vi "NMRvmefull5.vi"() -> ()   [LabVIEW 2013]
uses:
  <vilib>/Utility/file.llb/Read From Spreadsheet File (DBL).vi
  <vilib>/Analysis/NI_AALBase.lvlib
panel:
  in  "Real/quad Q curve":bool=TRUE
  out "Temperature (C)":dbl(graph)=26.0
  out "+3V supply":dbl=3.026 format="%_4g"
  out "Temp (C)":dbl=26.0 format="%_4g"
  in  "RemovePed":bool=TRUE
  in  "IF / LOG Det":bool
  in  "Q curve file":string="realback213.txt"
  out "File name 2":string="C:\\users\\plm\\Desktop\\rssmt\\realback213.txt"
  in  "AutoBaseline":bool=TRUE
  out "RF OK":bool=TRUE
  out "Peak area (V-MHz)":sgl=0.047548737 format="%.5f"
  in  "Gauss Fit":bool=TRUE
  out "NMR Graph + Fit":cluster{cluster{dbl, "Numeric":dbl}[]}[](graph)=[{[{212.6, "Numeric"=-0.023529166666666664}, {212.60999999999999, "Numeric"=0.005982291666645268}, {212.62, "Numeric"=0.0036937500000235666}, {212.63, "Numeric"=-0.001994791666664122}, {212.64, "Numeric"=0.00021666666664931725}, {212.65, "Numeric"=-0.006471874999975841}, {212.66, "Numeric"=0.00913958333333801}, {212.67, "Numeric"=-0.005548958333346967}, {212.68, "Numeric"=0.01206250000002431}, {212.69, "Numeric"=0.004273958333339739}, {212.7, "Numeric"=0.00948541666665629}, {212.71, "Numeric"=0.006996875000024064}, {212.72, "Numeric"=0.010408333333341034}, {212.73, "Numeric"=-0.0007802083333407752}, {212.74, "Numeric"=-0.0026687500000218346}, {212.75, "Numeric"=0.00804270833334196}, {212.76, "Numeric"=-0.005945833333338348}, {212.77, "Numeric"=0.006565624999982199}, {212.78, "Numeric"=-0.014122916666657513}, {212.79, "Numeric"=0.004488541666663723}, {212.8, "Numeric"=-0.0026000000000141266}, {212.81, "Numeric"=-0.01418854166665745}, {212.82, "Numeric"=0.003322916666665406}, {212.82999999999998, "Numeric"=-0.0057656250000106815}, {212.84, "Numeric"=0.005045833333342235}, {212.85, "Numeric"=0.00045729166666663755}, {212.85999999999999, "Numeric"=0.009268749999992144}, {212.87, "Numeric"=0.0015802083333415066}, {212.88, "Numeric"=-0.0008083333333325294}, {212.89, "Numeric"=0.006903124999994543}, {212.9, "Numeric"=0.006914583333340364}, {212.91, "Numeric"=0.019626041666667912}, {212.92, "Numeric"=0.017537499999996535}, {212.93, "Numeric"=0.03184895833333881}, {212.94, "Numeric"=0.042160416666667914}, {212.95, "Numeric"=0.08397187499999814}, {212.96, "Numeric"=0.14308333333333687}, {212.97, "Numeric"=0.2796947916666675}, {212.98, "Numeric"=0.4758062499999993}, {212.99, "Numeric"=0.4924177083333319}, {213.0, "Numeric"=0.3697291666666667}, {213.01, "Numeric"=0.32994062500000004}, {213.02, "Numeric"=0.3085520833333343}, {213.03, "Numeric"=0.25276354166666554}, {213.04, "Numeric"=0.2412750000000005}, {213.05, "Numeric"=0.2554864583333362}, {213.06, "Numeric"=0.23649791666666387}, {213.07, "Numeric"=0.26220937500000036}, {213.08, "Numeric"=0.21542083333333772}, {213.09, "Numeric"=0.17623229166666188}, {213.1, "Numeric"=0.10804374999999992}, {213.11, "Numeric"=0.0878552083333388}, {213.12, "Numeric"=0.07366666666665944}, {213.13, "Numeric"=0.06387812499999908}, {213.14000000000001, "Numeric"=0.05268958333333953}, {213.15, "Numeric"=0.0238010416666566}, {213.16, "Numeric"=0.04101249999999778}, {213.17000000000002, "Numeric"=0.044323958333339825}, {213.18, "Numeric"=0.04973541666665334}, {213.19, "Numeric"=0.01754687499999609}, {213.2, "Numeric"=0.013558333333339938}, {213.21, "Numeric"=0.01546979166664969}, {213.22, "Numeric"=-0.0050187500000060045}, {213.23, "Numeric"=0.006992708333339413}, {213.24, "Numeric"=-0.004495833333314304}, {213.25, "Numeric"=-0.004484375000008534}, {213.26, "Numeric"=-0.020372916666661543}, {213.27, "Numeric"=-0.013161458333313683}, {213.28, "Numeric"=-0.02475000000001141}, {213.29, "Numeric"=-0.009238541666662908}, {213.3, "Numeric"=-0.003027083333313468}, {213.31, "Numeric"=-0.009215625000014757}, {213.32, "Numeric"=0.007595833333335376}, {213.33, "Numeric"=-0.01389270833331363}, {213.34, "Numeric"=-0.0015812500000184572}, {213.35, "Numeric"=-0.02236979166666679}, {213.36, "Numeric"=-0.005258333333314221}, {213.37, "Numeric"=-0.01264687500002265}, {213.38, "Numeric"=0.0028645833333306244}, {213.39000000000001, "Numeric"=0.003176041666684711}, {213.4, "Numeric"=-0.012812500000027156}]}, {[{212.6, "Numeric"=8.849236916727226e-16}, {212.60999999999999, "Numeric"=4.394384601054511e-15}, {212.62, "Numeric"=2.0985812753655877e-14}, {212.63, "Numeric"=9.638046352087863e-14}, {212.64, "Numeric"=4.2568438081885237e-13}, {212.65, "Numeric"=1.8080977585312592e-12}, {212.66, "Numeric"=7.385698722155563e-12}, {212.67, "Numeric"=2.9013275083294973e-11}, {212.68, "Numeric"=1.0960677793739773e-10}, {212.69, "Numeric"=3.9821127664234395e-10}, {212.7, "Numeric"=1.3913140959130146e-09}, {212.71, "Numeric"=4.674899766090939e-09}, {212.72, "Numeric"=1.5106188854084262e-08}, {212.73, "Numeric"=4.6943233797290934e-08}, {212.74, "Numeric"=1.4028995801745716e-07}, {212.75, "Numeric"=4.0319547967580955e-07}, {212.76, "Numeric"=1.1143977110530282e-06}, {212.77, "Numeric"=2.9621036818992547e-06}, {212.78, "Numeric"=7.571741666412111e-06}, {212.79, "Numeric"=1.861344705003916e-05}, {212.8, "Numeric"=4.400411751348745e-05}, {212.81, "Numeric"=0.00010004498215640012}, {212.82, "Numeric"=0.00021874230998249162}, {212.82999999999998, "Numeric"=0.000459944854564812}, {212.84, "Numeric"=0.0009300669738067933}, {212.85, "Numeric"=0.0018086651440458608}, {212.85999999999999, "Numeric"=0.0033824984230175037}, {212.87, "Numeric"=0.0060834861572851085}, {212.88, "Numeric"=0.010522112315018461}, {212.89, "Numeric"=0.01750204636331994}, {212.9, "Numeric"=0.02799691729611715}, {212.91, "Numeric"=0.043069227921479894}, {212.92, "Numeric"=0.06371760543323779}, {212.93, "Numeric"=0.09065406723828814}, {212.94, "Numeric"=0.12403682153350193}, {212.95, "Numeric"=0.16321100973789646}, {212.96, "Numeric"=0.20653029346152152}, {212.97, "Numeric"=0.25133534099773286}, {212.98, "Numeric"=0.29414322257439385}, {212.99, "Numeric"=0.33105459459282993}, {213.0, "Numeric"=0.35832398627304507}, {213.01, "Numeric"=0.37298179077906635}, {213.02, "Numeric"=0.37336608536055516}, {213.03, "Numeric"=0.35943270442259634}, {213.04, "Numeric"=0.33276359115440546}, {213.05, "Numeric"=0.2962712447445919}, {213.06, "Numeric"=0.2536755960012569}, {213.07, "Numeric"=0.20888312896102842}, {213.08, "Numeric"=0.16541067237733806}, {213.09, "Numeric"=0.12596769348406162}, {213.1, "Numeric"=0.09225508542608185}, {213.11, "Numeric"=0.06497659379648092}, {213.12, "Numeric"=0.04401077886247676}, {213.13, "Numeric"=0.028667951127131407}, {213.14000000000001, "Numeric"=0.01795848697980128}, {213.15, "Numeric"=0.01081878077306337}, {213.16, "Numeric"=0.0062679046995669395}, {213.17000000000002, "Numeric"=0.003492222743199724}, {213.18, "Numeric"=0.0018711860703676314}, {213.19, "Numeric"=0.0009642008342720052}, {213.2, "Numeric"=0.0004778081108905347}, {213.21, "Numeric"=0.0002277062862031423}, {213.22, "Numeric"=0.00010435950496686319}, {213.23, "Numeric"=4.59964684274824e-05}, {213.24, "Numeric"=1.949631143558009e-05}, {213.25, "Numeric"=7.947232283822858e-06}, {213.26, "Numeric"=3.115407404336461e-06}, {213.27, "Numeric"=1.1744898726144466e-06}, {213.28, "Numeric"=4.258132708886193e-07}, {213.29, "Numeric"=1.4846517564983923e-07}, {213.3, "Numeric"=4.978121452820941e-08}, {213.31, "Numeric"=1.605247001264361e-08}, {213.32, "Numeric"=4.977986726313633e-09}, {213.33, "Numeric"=1.4845713971639958e-09}, {213.34, "Numeric"=4.2577869954237846e-10}, {213.35, "Numeric"=1.1743627334870057e-10}, {213.36, "Numeric"=3.1149858544759133e-11}, {213.37, "Numeric"=7.945941880801058e-12}, {213.38, "Numeric"=1.9492618235586696e-12}, {213.39000000000001, "Numeric"=4.598651068386541e-13}, {213.4, "Numeric"=1.0433408850441348e-13}]}]
  in  "Amp of Q curve":dbl=3.0 min=0.0 max=7.0 step=0.01 format="%_3f"
  in  "Subtract Q curve":bool=TRUE
  in  "Adjust Tune":bool
  out "Pedestal Offset":dbl(graph)=0.048295833333333406
  out "Pedestal Difference":dbl(graph)=0.004958333333337339
  out "# Good Spectra":i32=988
  in  "Quality cuts":bool=TRUE
  out "Pedestal OK":bool=TRUE
  out "Sweep #":i32=1000
  out "1st Sweep":bool
  out "ADC volts OK":bool=TRUE
  out "Peak Height Distribution":cluster{"Y":dbl[], "Y":dbl[]}[](graph)=[{"Y"=[0.3632886404655094, 0.363528262295063, 0.36376788412461664, 0.36400750595417025, 0.3642471277837239, 0.36448674961327754, 0.36472637144283115, 0.36496599327238477, 0.3652056151019384, 0.365445236931492, 0.3656848587610456, 0.3659244805905993, 0.3661641024201529, 0.3664037242497065, 0.36664334607926014, 0.36688296790881375, 0.36712258973836737, 0.367362211567921, 0.36760183339747465, 0.36784145522702827, 0.3680810770565819, 0.3683206988861355, 0.3685603207156891, 0.36879994254524273, 0.36903956437479635, 0.36927918620435, 0.36951880803390363, 0.36975842986345725, 0.36999805169301087, 0.3702376735225645, 0.3704772953521181, 0.3707169171816717, 0.3709565390112254, 0.371196160840779, 0.3714357826703326, 0.37167540449988623, 0.37191502632943985, 0.37215464815899346, 0.3723942699885471, 0.37263389181810075, 0.37287351364765436, 0.373113135477208, 0.3733527573067616, 0.3735923791363152, 0.3738320009658688, 0.37407162279542244, 0.3743112446249761, 0.37455086645452973, 0.37479048828408335, 0.37503011011363696, 0.3752697319431906, 0.3755093537727442, 0.3757489756022978, 0.3759885974318514, 0.3762282192614051, 0.3764678410909587, 0.3767074629205123, 0.37694708475006594, 0.37718670657961956, 0.3774263284091732, 0.3776659502387268, 0.37790557206828046, 0.3781451938978341, 0.3783848157273877, 0.3786244375569413, 0.3788640593864949, 0.37910368121604854, 0.37934330304560215, 0.3795829248751558, 0.37982254670470944, 0.38006216853426306, 0.38030179036381667, 0.3805414121933703, 0.3807810340229239, 0.3810206558524775, 0.3812602776820312, 0.3814998995115848, 0.3817395213411384, 0.38197914317069204, 0.38221876500024565, 0.38245838682979927, 0.3826980086593529, 0.38293763048890656, 0.38317725231846017, 0.3834168741480138, 0.3836564959775674, 0.383896117807121, 0.38413573963667463, 0.38437536146622825, 0.3846149832957819, 0.38485460512533554, 0.38509422695488915, 0.38533384878444277, 0.3855734706139964, 0.38581309244355, 0.3860527142731036, 0.3862923361026573, 0.3865319579322109, 0.3867715797617645, 0.38701120159131813], "Y"=[3.0, 0.0, 1.0, 2.0, 3.0, 1.0, 2.0, 3.0, 3.0, 0.0, 1.0, 4.0, 2.0, 4.0, 6.0, 3.0, 3.0, 5.0, 5.0, 4.0, 5.0, 4.0, 10.0, 3.0, 6.0, 7.0, 9.0, 14.0, 8.0, 13.0, 13.0, 13.0, 9.0, 16.0, 15.0, 18.0, 15.0, 17.0, 23.0, 24.0, 10.0, 18.0, 23.0, 18.0, 20.0, 17.0, 20.0, 19.0, 12.0, 21.0, 17.0, 21.0, 15.0, 24.0, 18.0, 21.0, 16.0, 17.0, 18.0, 14.0, 18.0, 23.0, 19.0, 13.0, 22.0, 10.0, 15.0, 14.0, 14.0, 9.0, 19.0, 14.0, 14.0, 11.0, 8.0, 5.0, 13.0, 8.0, 4.0, 13.0, 3.0, 7.0, 7.0, 3.0, 2.0, 3.0, 3.0, 2.0, 4.0, 2.0, 2.0, 3.0, 4.0, 4.0, 3.0, 1.0, 5.0, 3.0, 2.0, 3.0]}]
  in  "# of Sweeps":i32=1000
  out "Std Dev (V)":dbl=0.004671852680077797 format="%_2g"
  out "Peak mean (V)":dbl=0.37543357970562535 format="%_4g"
  out "Peak Height":dbl(graph)=0.375005560471768
  in  "Raw Data":bool=TRUE
  in  "Tank RF":bool=TRUE
  in  "IF Atten (dB)":i8 min=0 max=31 step=1
  in  "IFoffset (V)":dbl=-2.058603999999996 min=-4.0 max=4.0 step=0.001 format="%.4f"
  in  "Tune  (V)":dbl=0.6148999999999999 min=0.0 max=5.0 step=0.001 format="%.4f"
  in  "Hi / Lo IF Gain":bool
  out "Voltage Array":sgl[](array[numeric])=[0.5133, 0.5189, 0.4933, 0.4649, 0.445, 0.4168, 0.4115, 0.3765, 0.3744, 0.3475, 0.3342, 0.3138, 0.2999, 0.272, 0.254, 0.2492, 0.2203, 0.2185, 0.1841, 0.1896, 0.17, 0.1465, 0.1527, 0.1329, 0.1336, 0.1195, 0.1194, 0.1034, 0.0933, 0.0939, 0.0874, 0.0942, 0.0868, 0.0964, 0.1026, 0.1409, 0.1971, 0.3314, 0.5258, 0.5413, 0.4181, 0.3784, 0.3577, 0.3032, 0.2936, 0.3103, 0.2944, 0.3238, 0.2813, 0.247, 0.1843, 0.1702, 0.1627, 0.1602, 0.1569, 0.1365, 0.1628, 0.1758, 0.1915, 0.1702, 0.1777, 0.1917, 0.1839, 0.2092, 0.2116, 0.2261, 0.2253, 0.2482, 0.2529, 0.2853, 0.309, 0.3209, 0.3564, 0.3542, 0.3864, 0.3861, 0.4243, 0.4386, 0.4764, 0.4996, 0.5071] format="%.4f"
  in  "Invert Polarity":bool
  out "Pedestal Diff (V)":sgl=0.0049583334 format="%.3f"
  out "Peak amp (V)":sgl=0.37500557 format="%.3f"
  in  "Save Data to File":bool
  in  "RF Level (dBm)":dbl=-1.0 min=-10.0 max=1.0 step=0.1 format="%.2f"
  out "SMT error out":errorcluster
  out "Sample RMS (V)":dbl=0.013024691358024691 format="%.4f"
  in  "# Sample/step":i32=80 min=1 max=1000 step=100
  in  "Step Width (MHz)":dbl=0.01 min=0.0 max=1000.0 step=0.0005 format="%.4f"
  in  "Freq Span (MHz)":dbl=0.8 min=0.0 max=3000.0 step=0.1 format="%.3f"
  in  "Center Freq (MHz)":dbl=213.0 min=0.005 max=6000.0 step=0.1 format="%.3f"
  in  "Sweep Mode":u16(ring)=3 items=["Off", "Single", "Auto", "Step"]
  in  "GPIB Addr (28)":refnum<visa-resource-name>="GPIB0::28::INSTR"
  # "E1039 Prototype NMR Control Panel"
  # "Settings"
  # "D\nA\nC"
  # "R\nF\n\nG\nE\nN \n\n+\n\nI\nF"
  # "A\nD\nC"
  # "D\nA\nT\nA\n\n+\n\nA \nN\nA\nL\nY\nS\nI\nS"
  # "I\n/\nO"
  # "Results"
  # "A\nv\ne\nr\na\ng\ne"
  # "S\nw\ne\ne\np"
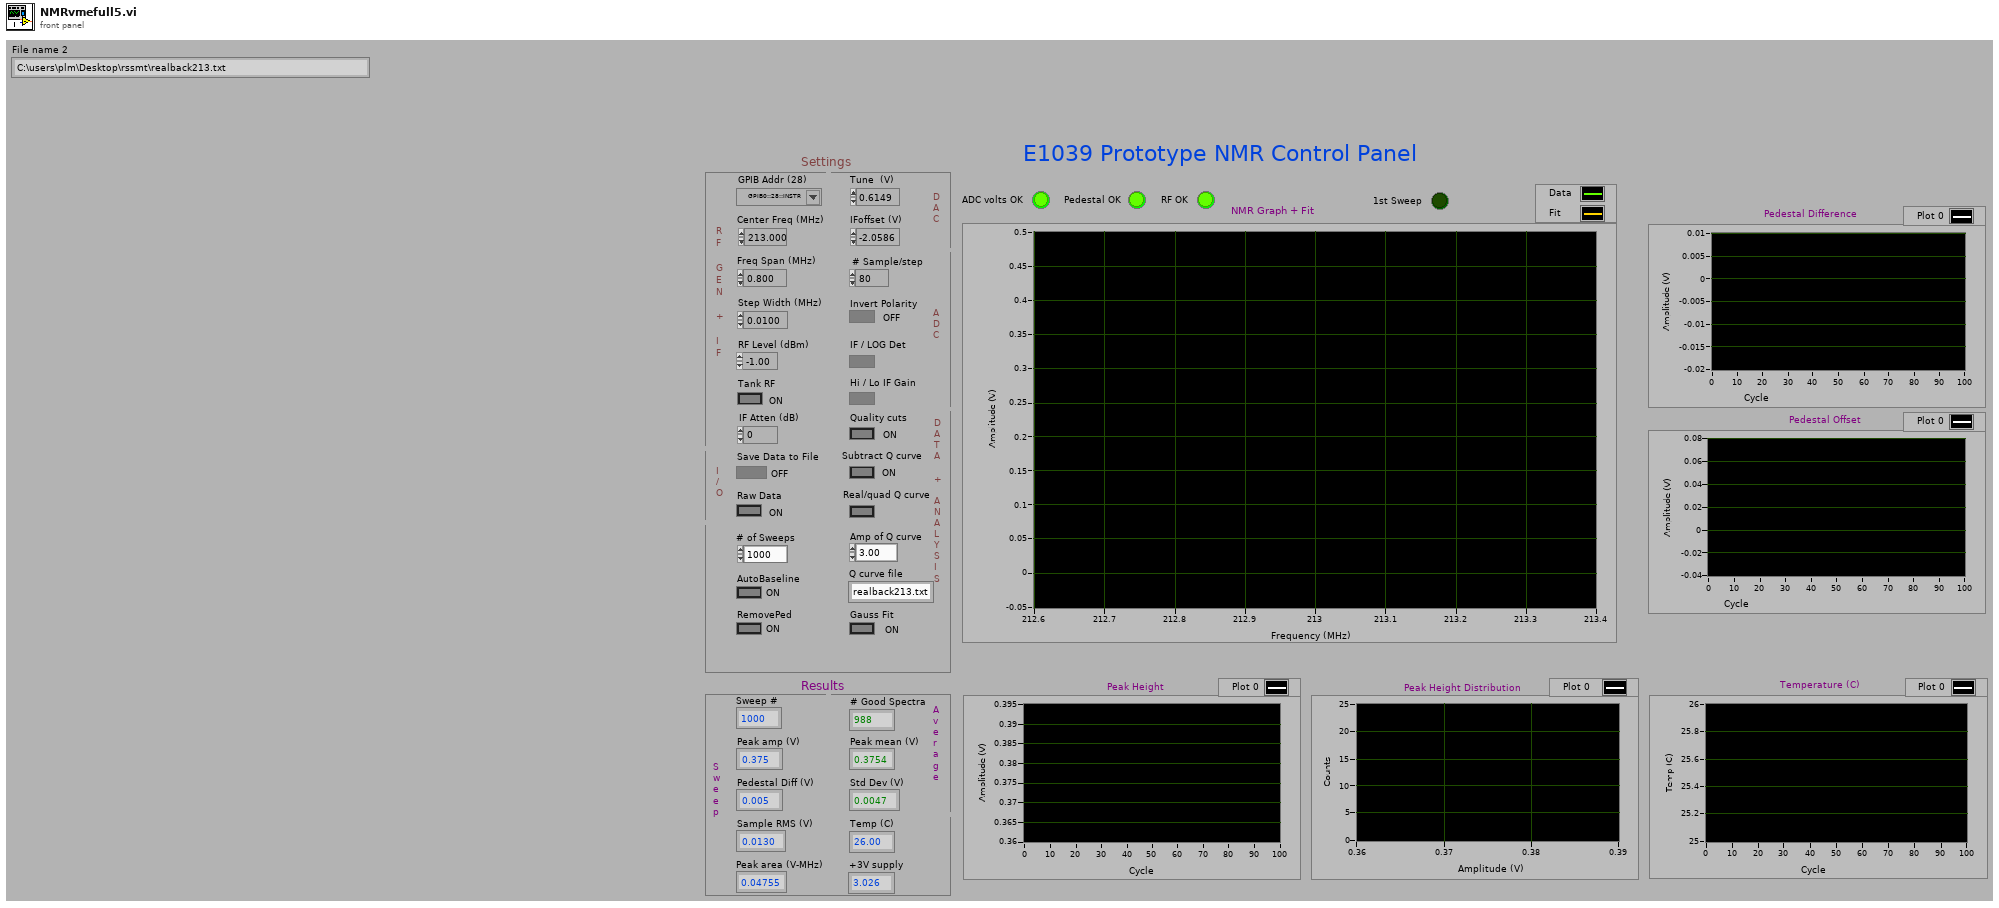
[diagram p1: front panel]
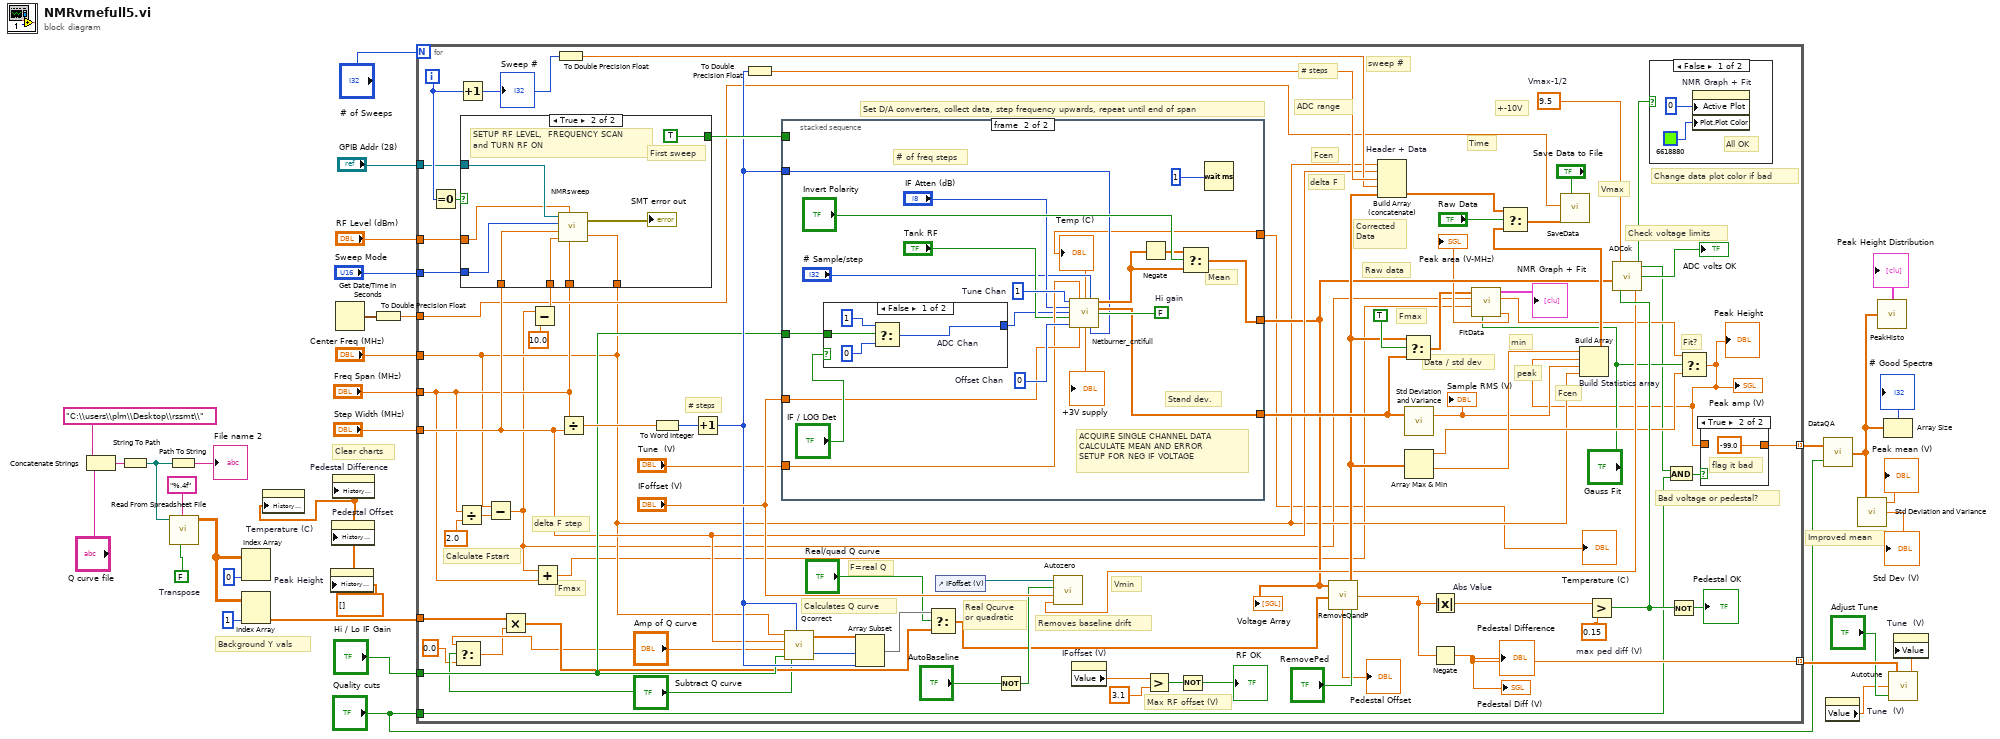
[diagram p0: block diagram]
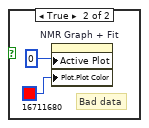
[diagram p2: hidden frame]
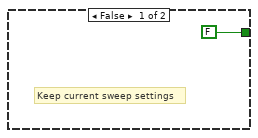
[diagram p4: hidden frame]
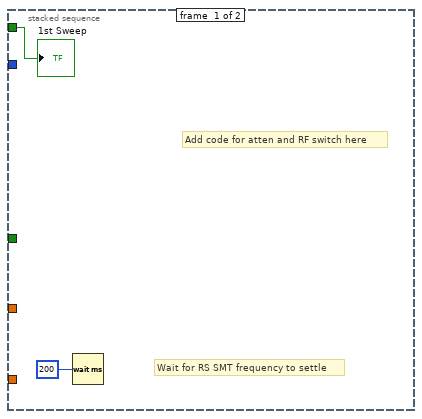
[diagram p5: hidden frame]
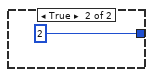
[diagram p6: hidden frame]
diagram:
  w9 = FALSE  # Transpose
  w1 = dbl[] []
  # "Background Y vals"
  # "Clear charts"
  # "Improved mean"
  n1 = Concatenate Strings "Concatenate Strings"("C:\\users\\plm\\Desktop\\rssmt\\", "Q curve file") -> (w12:string)
  n2 = String To Path(string=w12) -> (path=w8:path)
  n3 = Path To String(path=w8) -> (string=→"File name 2":string)
  n4 = call-poly <vilib>:"Read From Spreadsheet File.vi"("transpose (no:F)"=w9, "format (%.3f)"="%.4f", "file path (dialog if empty)"=w8) -> ("all rows"=w7:dbl[][])  [unwired: 4 in, 4 out]
  n5 = Index Array "Index Array"(array=w7, index (col)=0) -> ()  [unwired: 1 in, 1 out]
  n6 = Index Array(array=w7, index (col)=1) -> (element=w2:dbl[])  [unwired: 1 in]
  n7 = property on="Temperature (C)" class="WFChart (strict)"("History Data"=w1) -> ()  [unwired: 2 in, 2 out]
  n8 = property on="Peak Height" class="WFChart (strict)"("History Data"=w1) -> ()  [unwired: 2 in, 2 out]
  n9 = property on="Pedestal Offset" class="WFChart (strict)"("History Data"=w1) -> ()  [unwired: 2 in, 2 out]
  n10 = property on="Pedestal Difference" class="WFChart (strict)"("History Data"=w1) -> ()  [unwired: 2 in, 2 out]
  n11 = Get Date/Time In Seconds() -> (seconds since 1Jan1904=w14:timestamp)
  n12 = To Double Precision Float(number=w14) -> (double precision float=w13:dbl)
  n13 = for {
    N: "# of Sweeps" -> [_]
    tunnel: [w94] -> w29 mode=indexing
    tunnel: "Quality cuts" -> [w71]
    tunnel: [w77] -> w26 mode=indexing
    tunnel: "Center Freq (MHz)" -> [w58]
    tunnel: "Freq Span (MHz)" -> [w64]
    tunnel: "Step Width (MHz)" -> [w70]
    tunnel: "Sweep Mode" -> [w81]
    tunnel: "Hi / Lo IF Gain" -> [w80]
    tunnel: "GPIB Addr (28)" -> [w79]
    tunnel: "RF Level (dBm)" -> [w78]
    tunnel: w13 -> [w65]
    tunnel: w2 -> [w43]
    i -> [w92]
    w75 = 9.5  # Vmax-1/2
    w95 = 0.15  # max ped diff (V)
    # "F=real Q"
    # "Real Qcurve\nor quadratic"
    # "+-10V"
    # "Vmax"
    # "Change data plot color if bad"
    # "Max RF offset (V)"
    # "Fmax"
    # "Fit?"
    # "Fmax"
    # "Time"
    # "Vmin"
    # "min"
    # "peak"
    # "Raw data"
    # "Corrected\nData"
    # "Fcen"
    # "delta F"
    # "# steps"
    # "ADC range"
    # "sweep #"
    # "Fcen"
    # "Set D/A converters, collect data, step frequency upwards, repeat until end of span"
    # "Calculates Q curve"
    # "Removes baseline drift"
    # "Bad voltage or pedestal?"
    # "Check voltage limits"
    # "Data / std dev"
    # "# steps"
    # "Calculate Fstart"
    # "delta F step"
    n14 = Equal To 0?(x=w92) -> (x = 0?=w97:bool)
    n15 = Select(t="Amp of Q curve", s="Subtract Q curve", f=0.0) -> (s? t:f=w38:dbl)
    n16 = Divide(x=w64, y=sgl 2.0) -> (x/y=w108:dbl)
    n17 = Increment(x=w92) -> (x+1=w82:i32)
    "Sweep #" <- w82
    n18 = Subtract(x=w58, y=w108) -> (x-y=w53:dbl)
    n19 = Multiply(x=w43, y=w38) -> (x*y=w42:dbl[])
    n20 = Subtract(x=w53, y=10.0) -> (x-y=w106:dbl)
    n21 = case shown="True" w97 {
      tunnel: w106 -> [_ w126]
      tunnel: w70 -> [_ w124]
      tunnel: w58 -> [_ w123]
      tunnel: w64 -> [_ w125]
      tunnel: [FALSE TRUE] -> w96
      tunnel: w81 -> [_ w120]
      tunnel: w79 -> [_ w119]
      tunnel: w78 -> [_ w118]
      frame False {
        # "Keep current sweep settings"
      }
      frame True {
        # "First sweep"
        # "SETUP RF LEVEL,  FREQUENCY SCAN\nand TURN RF ON"
        n22 = call "NMRsweep.vi"("Center Freq (MHz)"=w123, "Freq Span (MHz)"=w125, "RF Level (dBm)"=w118, "Foffset (MHz)"=w126, "Step Width (MHz)"=w124, "Sweep Mode"=w120, "GPIB Addr (28)"=w119) -> ("error out"=→"SMT error out":errorcluster)
      }
    }
    n23 = Add(x=w53, y=w64) -> (x+y=w52:dbl)
    n24 = To Double Precision Float(number=w82) -> (double precision float=w83:dbl)
    n25 = Divide(x=w64, y=w70) -> (x/y=w110:dbl)
    n26 = To Word Integer(number=w110) -> (16bit integer=w107:i16)
    n27 = Increment(x=w107) -> (x+1=w86:i16)
    n28 = To Double Precision Float(number=w86) -> (double precision float=w85:dbl)
    n29 = stacked-sequence {
      tunnel: [_ w134] -> w100
      tunnel: [_ w146] -> w68
      tunnel: w86 -> [_ w131]
      tunnel: "IFoffset (V)" -> [_ w141]
      tunnel: w80 -> [_ w144]
      tunnel: w96 -> [w127 _]
      tunnel: "Tune  (V)" -> [_ w139]
      tunnel: [_ w129] -> w34
      frame #0 {
        # "Add code for atten and RF switch here"
        # "Wait for RS SMT frequency to settle"
        n30 = Wait (ms)(milliseconds to wait=200) -> ()  [unwired: 1 out]
        "1st Sweep" <- w127
      }
      frame #1 {
        w136 = FALSE  # Hi gain
        w142 = 0  # Offset Chan
        w140 = 1  # Tune Chan
        # "Stand dev."
        # "Mean"
        # "ACQUIRE SINGLE CHANNEL DATA\nCALCULATE MEAN AND ERROR\nSETUP FOR NEG IF VOLTAGE"
        # "# of freq steps"
        n31 = case shown="False" "IF / LOG Det" {
          tunnel: w144 -> [w152 _]
          tunnel: [w149 2] -> w133
          frame False {
            n32 = Select "ADC Chan"(t=1, s=w152, f=0) -> (s? t:f=w149:i32)
          }
          frame True {
          }
        }
        n33 = call "Netburner_cntlfull.vi"("Tune DAC"=w140, "Tune Volt"=w139, "# Data"="# Sample/step", "IF Atten (dB)"="IF Atten (dB)", "NMR ADC"=w133, "Hi Gain"=w136, "Tank RF"="Tank RF", "Offset DAC"=w142, "Offset Volt"=w141, "# f steps"=w131) -> ("Temp (C)"=w129:dbl, "ADC value"=w135:dbl[], "ADC error"=w134:dbl[], "Volts"=→"+3V supply":dbl)  [unwired: 2 out]
        "Temp (C)" <- w129
        n34 = Negate(x=w135) -> (-x=w145:dbl[])
        n35 = Select(t=w145, s="Invert Polarity", f=w135) -> (s? t:f=w146:dbl[])
        n36 = Wait (ms)(milliseconds to wait=1) -> ()  [unwired: 1 out]
      }
    }
    "Voltage Array" <- w68
    "Temperature (C)" <- w34
    n37 = call "Qcorrect.vi"("Subtract Q curve"="Subtract Q curve", "Nstep"=w86, "IF or Log"=w80, "Amp of Q curve"="Amp of Q curve", "Step Width (MHz)"=w70, "Center Freq (MHz)"=w58) -> ("Start"=w101:i32, "Array"=w102:dbl[])
    n38 = Array Subset "Array Subset"(array=w102, index=w101, length=w86) -> (w46:dbl[])
    n39 = Select(t=w46, s="Real/quad Q curve", f=w42) -> (s? t:f=w45:dbl[])
    n40 = control-ref of="IFoffset (V)"() -> (w74:refnum<vi>)
    n41 = Not(x="AutoBaseline") -> (.not. x?=w47:bool)
    n42 = property on="IFoffset (V)" class="DigNum (strict)"() -> ("Value"=w62:dbl)  [unwired: 2 in, 2 out]
    n43 = Greater?(x=w62, y=3.1) -> (0:w60:bool)
    n44 = Not(x=w60) -> (.not. x?=→"RF OK":bool)
    n45 = call "RemoveQandP.vi"("Subtract Ped?"="RemovePed", "Qcurve"=w45, "Raw data"=w68) -> ("Ped L-R"=w88:dbl, "Corrected data"=w84:dbl[], "Ped Offfset"=→"Pedestal Offset":dbl)
    n46 = Build Array (concatenate) "Header + Data"(w58, w70, w85, w83, w84) -> (w87:dbl[])
    n47 = Select(t=w84, s=TRUE, f=w100) -> (s? t:f=w54:dbl[])
    n48 = call <vilib>:"Std Deviation and Variance.vi"("X"=w100) -> ("mean"=w69:dbl)  [unwired: 1 in, 2 out]
    "Sample RMS (V)" <- w69
    n49 = Array Max & Min(array=w84) -> (max value=w63:dbl, min value=w99:dbl)  [unwired: 2 out]
    n50 = Absolute Value "Abs Value"(x=w88) -> (abs(x)=w90:dbl)
    n51 = Negate(x=w88) -> (-x=w77:dbl)
    "Pedestal Diff (V)" <- w77
    "Pedestal Difference" <- w77
    n52 = call "FitData.vi"("Fit?"="Gauss Fit", "Fmax"=w52, "Fmin"=w53, "Yarray"=w54) -> ("Peak Area (V-MHz)"=→"Peak area (V-MHz)":dbl, "Amplitude (V)"=w56:dbl, "NMR Graph + Fit"=→"NMR Graph + Fit":cluster{cluster{dbl, "Numeric":dbl}[]}[])  [unwired: 2 out]
    n53 = Greater?(x=w90, y=w95) -> (0:w76:bool)
    n54 = call "ADCok.vi"("PedOK"=w76, "Array"=w68, "Vmax-1/2"=w75) -> ("Vmin"=w73:dbl, "ADC voltages OK"=→"ADC volts OK":bool, "Allok"=w50:bool)
    n55 = call "Autozero.vi"("Vmin (V)"=w73, "IFoffset (V)"="IFoffset (V)", "IF or Log"=w47, "reference"=w74) -> ()
    n56 = case shown="False" w50 {
      frame False {
        # "All OK"
        n57 = property on="NMR Graph + Fit" class="XYGraph (strict)"("Active Plot"=0, "Plot.Plot Color"=u32 6618880) -> ()  [unwired: 2 in, 2 out]
      }
      frame True {
        # "Bad data"
        n58 = property on="NMR Graph + Fit" class="XYGraph (strict)"("Active Plot"=0, "Plot.Plot Color"=u32 16711680) -> ()  [unwired: 2 in, 2 out]
      }
    }
    n59 = And(x=w50, y=w71) -> (x .and. y?=w91:bool)
    n60 = Not(x=w76) -> (.not. x?=→"Pedestal OK":bool)
    n61 = Select(t=w56, s="Gauss Fit", f=w63) -> (s? t:f=w49:dbl)
    "Peak amp (V)" <- w49
    "Peak Height" <- w49
    n62 = Build Array "Build Statistics array"(w99, w49, w69, w58) -> (w105:dbl[])
    n63 = Select(t=w87, s="Raw Data", f=w105) -> (s? t:f=w66:dbl[])
    n64 = call "SaveData.vi"("Array"=w66, "Save Data to File"="Save Data to File", "Ext time (sec)"=w65) -> ()  [unwired: 1 out]
    n65 = case shown="True" w91 {
      tunnel: [w115 -99.0] -> w94
      tunnel: w49 -> [w115 _]
      frame False {
        # "Data OK"
      }
      frame True {
        # "flag it bad"
      }
    }
  }
  n66 = call "DataQA.vi"("Quality cuts"="Quality cuts", "Data In"=w29) -> ("Data Out"=w28:dbl[])
  n67 = property on="Tune  (V)" class="DigNum (strict)"() -> ("Value"=w17:dbl)  [unwired: 2 in, 2 out]
  n68 = call <vilib>:"Std Deviation and Variance.vi"("X"=w28) -> ("mean"=→"Peak mean (V)":dbl, "standard deviation"=→"Std Dev (V)":dbl)  [unwired: 1 in, 1 out]
  n69 = call "PeakHisto.vi"("Data Out"=w28) -> ("XY Graph"=→"Peak Height Distribution":cluster{"Y":dbl[], "Y":dbl[]}[])
  n70 = Array Size(array=w28) -> (size(s)=→"# Good Spectra":i32)
  n71 = call "Autotune.vi"("Adjust Tune"="Adjust Tune", "Tune Vin"=w17, "Pedestal Diff"=w26) -> ("Tune Vout"=w16:dbl)
  n72 = property on="Tune  (V)" class="DigNum (strict)"("Value"=w16) -> ()  [unwired: 2 in, 2 out]
